vi "demo_sinanju.vi"() -> ()   [LabVIEW 2017]
panel:
  in  "输入 3":string
  in  "t 2":sgl
  in  "d":sgl
  in  "t":sgl
  in  "z1":sgl
  in  "y1":sgl
  in  "x1":sgl
  out "值 4":sgl
  out "值 2":sgl
  out "值 3":sgl
  out "值":sgl
  in  "port":u16=1234
  in  "ip":string="192.168.1.44"
  in  "name":string="MRX-T4"
  out "读取缓冲区":string
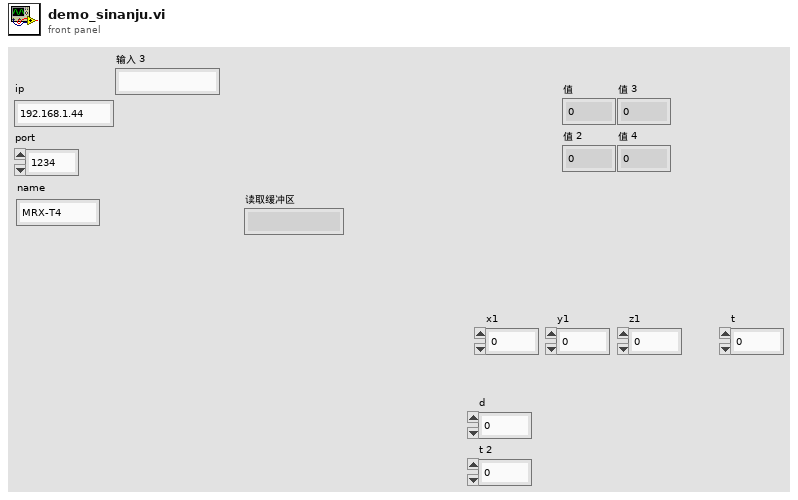
[diagram p1: front panel]
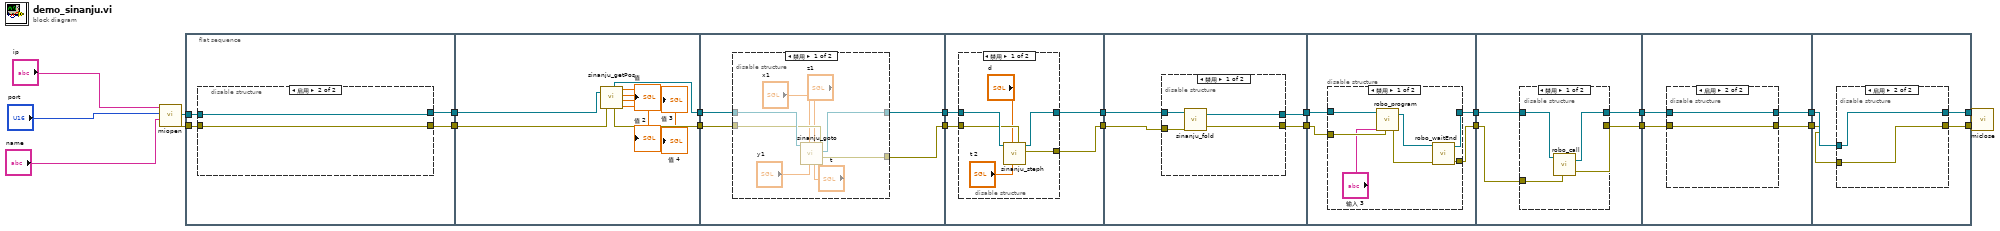
[diagram p0: block diagram]
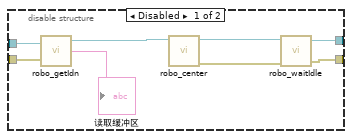
[diagram p2: hidden frame]
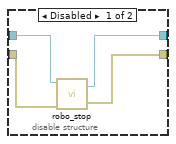
[diagram p8: hidden frame]
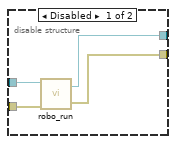
[diagram p9: hidden frame]
diagram:
  n1 = call "miopen.vi"("name"="name", "port"="port", "ip"="ip") -> ("错误输出"=w22:errorcluster, "VISA资源名称输出"=w23:refnum<visa-resource-name>)  [unwired: 1 in]
  n2 = flat-sequence {
    tunnel: w23 -> [w27]
    tunnel: w22 -> [w26]
    tunnel: [w25] -> w16
    tunnel: [w24] -> w15
    tunnel: w16 -> [w45]
    tunnel: w15 -> [w43]
    tunnel: [w44] -> w14
    tunnel: [w42] -> w13
    tunnel: w14 -> [w49]
    tunnel: w13 -> [w48]
    tunnel: [w47] -> w12
    tunnel: [w46] -> w11
    tunnel: w12 -> [w63]
    tunnel: w11 -> [w62]
    tunnel: [w61] -> w10
    tunnel: [w60] -> w9
    tunnel: w10 -> [w75]
    tunnel: w9 -> [w74]
    tunnel: [w73] -> w8
    tunnel: [w72] -> w7
    tunnel: w8 -> [w85]
    tunnel: w7 -> [w84]
    tunnel: [w83] -> w6
    tunnel: [w82] -> w5
    tunnel: w6 -> [w98]
    tunnel: w5 -> [w97]
    tunnel: [w96] -> w4
    tunnel: [w95] -> w3
    tunnel: w4 -> [w108]
    tunnel: w3 -> [w107]
    tunnel: [w106] -> w2
    tunnel: [w105] -> w1
    tunnel: [w115] -> w17
    tunnel: [w116] -> w18
    tunnel: w2 -> [w118]
    tunnel: w1 -> [w117]
    frame #0 {
      n3 = disable-structure shown="启用" {
        disable-tunnel: w27 -> [w34 w37]
        disable-tunnel: w26 -> [w33 w36]
        disable-tunnel: [w29 w37] -> w25
        disable-tunnel: [w28 w36] -> w24
        frame Disabled {
          n4 = call "robo_getIdn.vi"("VISA资源名称"=w34, "错误输入（无错误）"=w33) -> ("VISA资源名称输出"=w32:refnum<visa-resource-name>, "读取缓冲区"=→"读取缓冲区":string)  [unwired: 1 out]
          n5 = call "robo_center.vi"("VISA资源名称"=w32) -> ("错误输出"=w30:errorcluster, "VISA资源名称输出"=w31:refnum<visa-resource-name>)  [unwired: 3 in]
          n6 = call "robo_waitIdle.vi"("错误输入（无错误）"=w30, "VISA资源名称"=w31) -> ("错误输出"=w28:errorcluster, "VISA资源名称输出"=w29:refnum<visa-resource-name>)  [unwired: 2 in, 1 out]
        }
        frame Enabled {
        }
      }
    }
    frame #1 {
      n7 = call "sinanju_getPos.vi"("VISA资源名称"=w45, "错误输入（无错误）"=w43) -> ("VISA资源名称输出"=w44:refnum<visa-resource-name>, "错误输出"=w42:errorcluster, "值"=→"值":sgl, "值 2"=→"值 2":sgl, "值 3"=→"值 3":sgl, "值 4"=→"值 4":sgl)
    }
    frame #2 {
      n8 = disable-structure shown="禁用" {
        disable-tunnel: w49 -> [w57 w59]
        disable-tunnel: w48 -> [w56 w58]
        disable-tunnel: [w55 w59] -> w47
        disable-tunnel: [w54 w58] -> w46
        frame Disabled {
          n9 = call "sinanju_goto.vi"("错误输入（无错误）"=w56, "t"="t", "z1"="z1", "y1"="y1", "x1"="x1", "VISA资源名称"=w57) -> ("错误输出"=w54:errorcluster, "VISA资源名称输出"=w55:refnum<visa-resource-name>)  [unwired: 4 in]
        }
        frame Enabled {
        }
      }
    }
    frame #3 {
      n10 = disable-structure shown="禁用" {
        disable-tunnel: w63 -> [w69 w71]
        disable-tunnel: w62 -> [w68 w70]
        disable-tunnel: [w65 w71] -> w61
        disable-tunnel: [w64 w70] -> w60
        frame Disabled {
          n11 = call "sinanju_steph.vi"("错误输入（无错误）"=w68, "t"="t 2", "d"="d", "VISA资源名称"=w69) -> ("错误输出"=w64:errorcluster, "VISA资源名称输出"=w65:refnum<visa-resource-name>)  [unwired: 6 in]
        }
        frame Enabled {
        }
      }
    }
    frame #4 {
      n12 = disable-structure shown="禁用" {
        disable-tunnel: w75 -> [w79 w81]
        disable-tunnel: w74 -> [w78 w80]
        disable-tunnel: [w77 w81] -> w73
        disable-tunnel: [w76 w80] -> w72
        frame Disabled {
          n13 = call "sinanju_fold.vi"("错误输入（无错误）"=w78, "VISA资源名称"=w79) -> ("错误输出"=w76:errorcluster, "VISA资源名称输出"=w77:refnum<visa-resource-name>)  [unwired: 2 in]
        }
        frame Enabled {
        }
      }
    }
    frame #5 {
      n14 = disable-structure shown="禁用" {
        disable-tunnel: w85 -> [w92 w94]
        disable-tunnel: w84 -> [w91 w93]
        disable-tunnel: [w87 w94] -> w83
        disable-tunnel: [w86 w93] -> w82
        frame Disabled {
          n15 = call "robo_program.vi"("VISA资源名称"=w92, "输入 3"="输入 3", "错误输入（无错误）"=w91) -> ("VISA资源名称输出"=w89:refnum<visa-resource-name>, "错误输出"=w88:errorcluster)  [unwired: 2 in]
          n16 = call "robo_waitEnd.vi"("VISA资源名称"=w89, "错误输入（无错误）"=w88) -> ("VISA资源名称输出"=w87:refnum<visa-resource-name>, "错误输出"=w86:errorcluster)  [unwired: 3 in, 1 out]
        }
        frame Enabled {
        }
      }
    }
    frame #6 {
      n17 = disable-structure shown="禁用" {
        disable-tunnel: w98 -> [w102 w104]
        disable-tunnel: w97 -> [w101 w103]
        disable-tunnel: [w100 w104] -> w96
        disable-tunnel: [w99 w103] -> w95
        frame Disabled {
          n18 = call "robo_call.vi"("错误输入（无错误）"=w101, "VISA资源名称"=w102) -> ("错误输出"=w99:errorcluster, "VISA资源名称输出"=w100:refnum<visa-resource-name>)  [unwired: 4 in]
        }
        frame Enabled {
        }
      }
    }
    frame #7 {
      n19 = disable-structure shown="启用" {
        disable-tunnel: w108 -> [w112 w114]
        disable-tunnel: w107 -> [w111 w113]
        disable-tunnel: [w110 w114] -> w106
        disable-tunnel: [w109 w113] -> w105
        frame Disabled {
          n20 = call "robo_stop.vi"("错误输入（无错误）"=w111, "VISA资源名称"=w112) -> ("错误输出"=w109:errorcluster, "VISA资源名称输出"=w110:refnum<visa-resource-name>)  [unwired: 2 in]
        }
        frame Enabled {
        }
      }
    }
    frame #8 {
      n21 = disable-structure shown="启用" {
        disable-tunnel: w118 -> [w122 w124]
        disable-tunnel: w117 -> [w121 w123]
        disable-tunnel: [w120 w124] -> w116
        disable-tunnel: [w119 w123] -> w115
        frame Disabled {
          n22 = call "robo_run.vi"("错误输入（无错误）"=w121, "VISA资源名称"=w122) -> ("错误输出"=w119:errorcluster, "VISA资源名称输出"=w120:refnum<visa-resource-name>)  [unwired: 2 in]
        }
        frame Enabled {
        }
      }
    }
  }
  n23 = call "miclose.vi"("错误输入（无错误）"=w17, "VISA资源名称"=w18) -> ()  [unwired: 1 out]
